vi "Kontroll Interferent Beschreibung Tabelle.vi"(4 "Sprachliste":string[][](array[string]), 6 "MFC-auswahl":T1 items=["MFC 2", "MFC 3", "MFC 4", "MFC 5"], 10 "Table Header":string[](array[string]), 11 "TestKonfig":T2 {"TestKonfig Interferent"."Gasflasche MFC3" items=["----"=10000, "IAG NH3 3000"=0, "IAG NH3 200"=1, "IAG NH3 2000"=2, "IAG MG"=3, "IAG O2"=4]; "TestKonfig Interferent"."Gasflasche MFC2" items=["----"=10000, "IAG NH3 3000"=0, "IAG NH3 200"=1, "IAG NH3 2000"=2, "IAG MG"=3, "IAG O2"=4]; "TestKonfig Interferent"."Eingangs Konzentration MFC1" min=0.0; "TestKonfig Interferent"."Ausgangs Konzentration MFC1" min=0.0; "TestKonfig Interferent"."MFC2" items=["MFC 2", "MFC 3", "MFC 4", "MFC 5"]; "TestKonfig Interferent"."MFC3" items=["MFC 2", "MFC 3", "MFC 4", "MFC 5"]; "TestKonfig Interferent"."Ausgangs Konzentration MFC3" min=0.0; "TestKonfig Interferent"."Eingangs Konzentration MFC3" min=0.0; "TestKonfig Interferent"."Ausgangs Konzentration MFC2" min=0.0; "TestKonfig Interferent"."Eingangs Konzentration MFC2" min=0.0; "TestKonfig H2O"."HovaCAL Temperature" format="%.2f"; "TestKonfig H2O"."HovaCAL Flow Input Cluster"."HovaCAL Flow Input Cluster" format="%.2f"; "TestKonfig H2O"."Eingangs Konzentration:" min=0.0; "TestKonfig H2O"."zusätzliche Zeitdauer Erster Punkt" min=30 step=1 format="%#_5g"; "TestKonfig H2O"."Zeitdauer Stufen" format="%#_5g"; "TestKonfig H2O"."Max Fehler" format="%#_5g"; "TestKonfig H2O"."Anzahl Stufen" format="%#_5g"; "TestKonfig H2O"."Modus" items=["Messen", "CG zu Entnahmestelle"]}) -> (3 "Tabelle":string[][](array[string]))   [LabVIEW 2020, in "EPA 1065.lvlib" / "HovaCAL Interference verificaton.lvlib"]
uses:
  HovaCAL Interference verificaton.lvlib
  TestKonfig.ctl
  TestKonfig H2O.ctl
  Modus.ctl
  Linearisierung V2/SpanEinstellungen/Einheit.ctl
  Linearisierung V2/Gasteiler/Stufen Tabelle.ctl
  Linearisierung V2/Gasteiler/HovaCAL_Interface/Controls/Flow Einstellung.ctl
  Linearisierung V2/Gasteiler/HovaCAL_Interface/Controls/Temp Sollwerte Anzeige.ctl
  TestKonfig Interferents.ctl
  MFCAuswahl.ctl
  Seiten/System Einstellungen V2/Gasflasche Auswahl.ctl
  Sprachverwaltung/Sprachverwaltung.lvlib
  Linearisierung V2/SpanEinstellungen/SpanEinstellungen.lvlib
  Linearisierung V2/Gasteiler/Gasteiler.lvlib
  Linearisierung V2/Gasteiler/HovaCAL_Interface/Controls/Controls.lvlib
  Seiten/System Einstellungen V2/System Einstellungen V2.lvlib
panel:
  # "sec"
  # "%"
  # "sec"
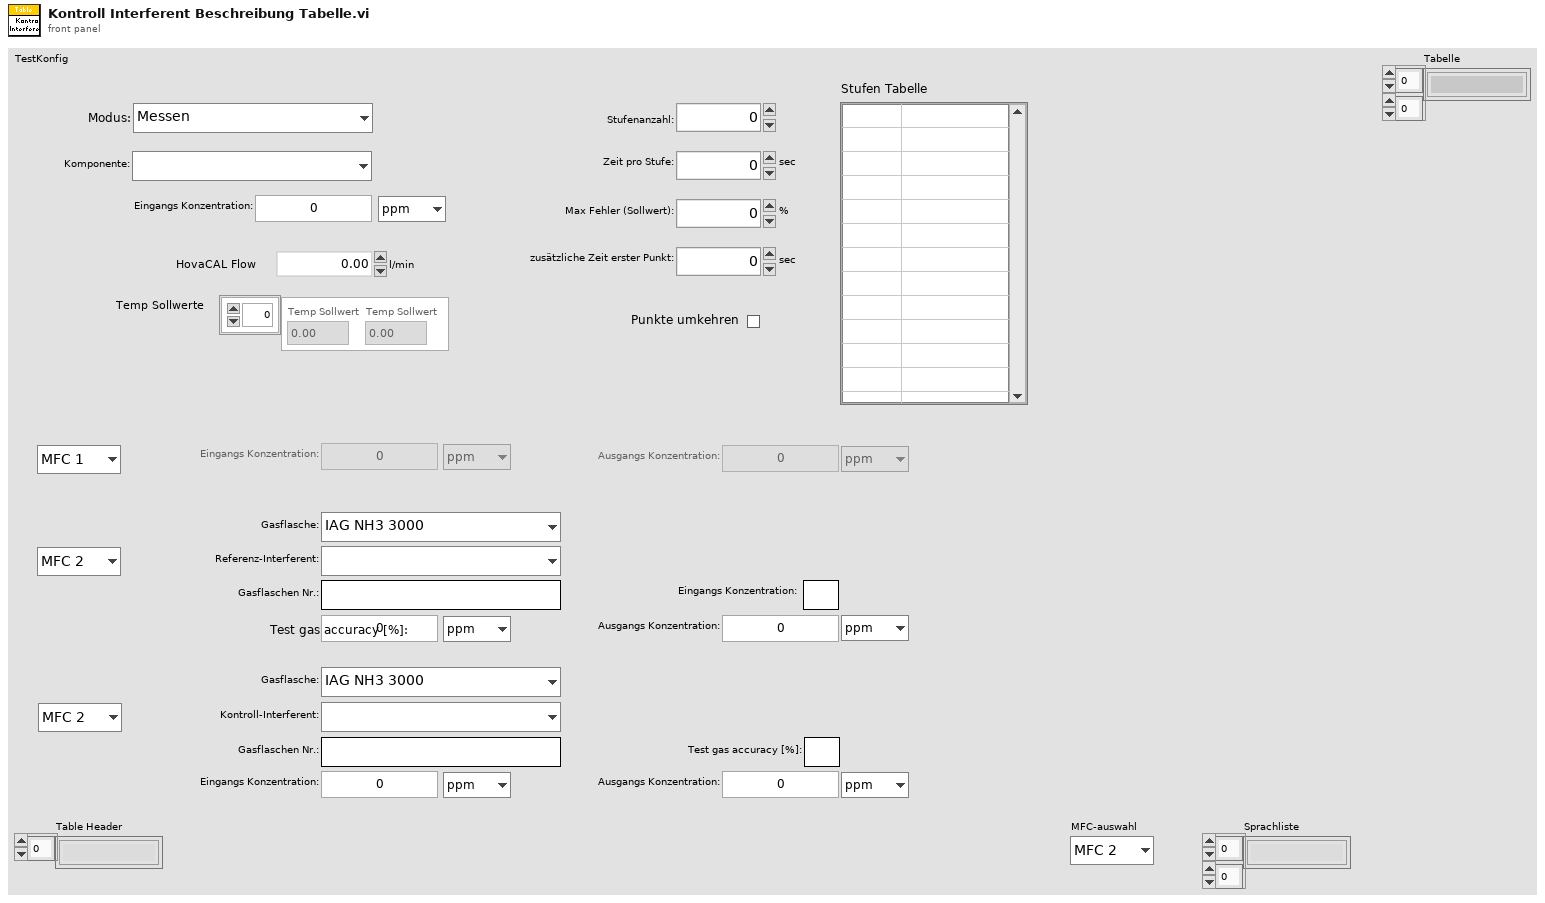
[diagram p1: front panel]
types:
  T1 = typedef "EPA 1065.lvlib/HovaCAL Interference verificaton.lvlib/MFCAuswahl.ctl" = u16
  T2 = typedef "EPA 1065.lvlib/HovaCAL Interference verificaton.lvlib/TestKonfig.ctl" = cluster{"TestKonfig H2O":T3, "TestKonfig Interferent":T9}
  T3 = typedef "EPA 1065.lvlib/HovaCAL Interference verificaton.lvlib/TestKonfig H2O.ctl" = cluster{"Modus":T4, "Komponente:":u16, "Eingangs Konzentration:":dbl, "Einheit":T5, "Anzahl Stufen":sgl, "Zeitdauer Stufen":sgl, "Max Fehler":sgl, "zusätzliche Zeitdauer Erster Punkt":sgl, "Punkte umkehren":bool, "Stufen Tabelle":T6, "HovaCAL Flow Input Cluster":T7, "HovaCAL Temperature":T8}
  T4 = typedef "EPA 1065.lvlib/HovaCAL Interference verificaton.lvlib/Modus.ctl" = u16
  T5 = typedef "Linearisierung v2.lvlib/SpanEinstellungen.lvlib/Einheit.ctl" = enum16{"ppm", "%"}
  T6 = typedef "Linearisierung v2.lvlib/Gasteiler.lvlib/Stufen Tabelle.ctl" = string[][]
  T7 = typedef "Linearisierung v2.lvlib/Gasteiler.lvlib/HovaCAL_Interface.lvlib/Controls.lvlib/Flow Einstellung.ctl" = cluster{"HovaCAL Flow Input Cluster":dbl}
  T8 = typedef "Linearisierung v2.lvlib/Gasteiler.lvlib/HovaCAL_Interface.lvlib/Controls.lvlib/Temp Sollwerte Anzeige.ctl" = dbl[]
  T9 = typedef "EPA 1065.lvlib/HovaCAL Interference verificaton.lvlib/TestKonfig Interferents.ctl" = cluster{"MFC1":enum16{"MFC 1"}, "Eingangs Konzentration MFC1":dbl, "Einheit MFC1 Eingang":T5, "Ausgangs Konzentration MFC1":dbl, "Einheit MFC1 Ausgang":T5, "MFC2":T1, "Referenz-Interferent:":u16, "Gasflaschen Nr MFC2":string, "Accuracy MFC2":string, "Eingangs Konzentration MFC2":dbl, "Einheit MFC2 Eingang":T5, "Ausgangs Konzentration MFC2":dbl, "Einheit MFC2 Ausgang":T5, "MFC3":T1, "Kontroll-Interferent:":u16, "Gasflaschen Nr MFC3":string, "Accuracy MFC3":string, "Eingangs Konzentration MFC3":dbl, "Einheit MFC3 Eingang":T5, "Ausgangs Konzentration MFC3":dbl, "Einheit MFC3 Ausgang":T5, "Gasflasche MFC2":T10, "Gasflasche MFC3":T10}
  T10 = typedef "System Einstellungen V2.lvlib/Gasflasche Auswahl.ctl" = u16
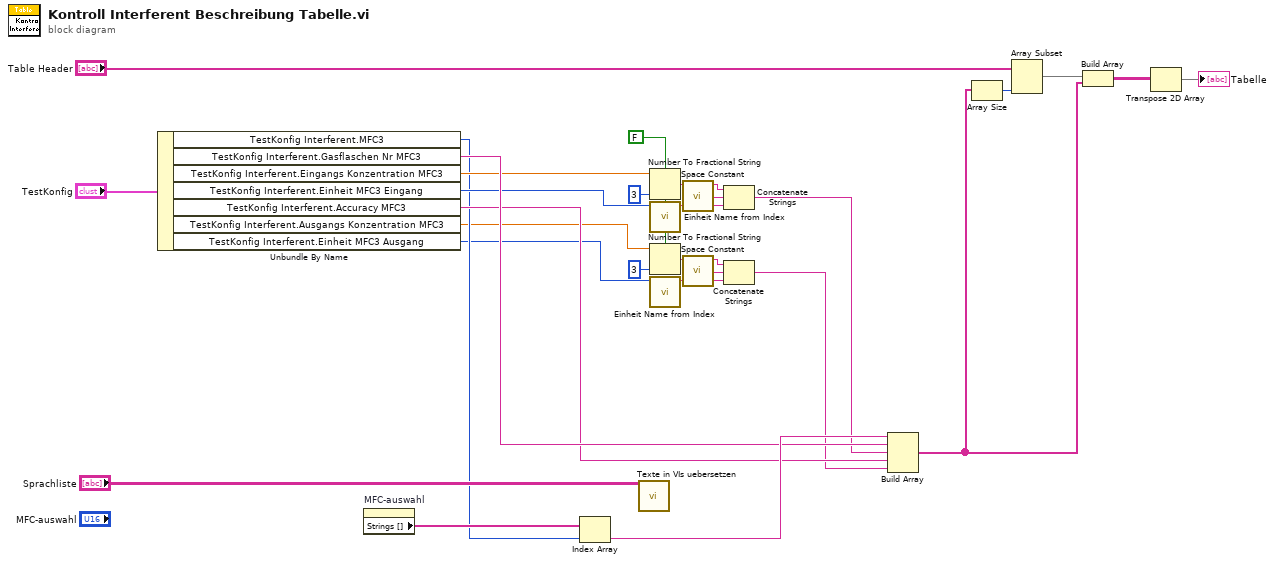
[diagram p0: block diagram]
diagram:
  w8 = FALSE ("Systemdezimalzeichen verwenden (T)")
  n1 = Unbundle By Name("TestKonfig") -> ("TestKonfig Interferent.MFC3"=w13:T1, "TestKonfig Interferent.Gasflaschen Nr MFC3"=w18:string, "TestKonfig Interferent.Eingangs Konzentration MFC3"=w17:dbl, "TestKonfig Interferent.Einheit MFC3 Eingang"=w15:T5, "TestKonfig Interferent.Accuracy MFC3"=w14:string, "TestKonfig Interferent.Ausgangs Konzentration MFC3"=w7:dbl, "TestKonfig Interferent.Einheit MFC3 Ausgang"=w6:T5)
  n2 = property on="MFC-auswahl" class="Ring (strikt)"() -> ("Strings []"=w20:string[])  [unwired: 2 in, 2 out]
  n3 = Index Array(array=w20, index=w13) -> (element=w19:string)
  n4 = call "Texte in VIs uebersetzen.vi"("Sprachliste"="Sprachliste") -> ()  [unwired: 10 in, 5 out]
  n5 = Number To Fractional String(use system decimal point (T)=w8, number=w17, precision (6)=i16 3 ("Genauigkeit (6)")) -> (F-format string=w23:string)  [unwired: 1 in]
  n6 = call "Einheit Name from Index.vi"("EinheitIndex"=w15) -> ("EinheitName"=w24:string)  [unwired: 10 in]
  n7 = Number To Fractional String(use system decimal point (T)=w8, number=w7, precision (6)=i16 3 ("Genauigkeit (6)")) -> (F-format string=w11:string)  [unwired: 1 in]
  n8 = call "Einheit Name from Index.vi"("EinheitIndex"=w6) -> ("EinheitName"=w10:string)  [unwired: 10 in]
  n9 = call <vilib>:"Space Constant.vi"() -> ("String"=w22:string)
  n10 = call <vilib>:"Space Constant.vi"() -> ("String"=w12:string)
  n11 = Concatenate Strings(w23, w22, w24) -> (w16:string)
  n12 = Concatenate Strings(w11, w12, w10) -> (w5:string)
  n13 = Build Array(w19, w18, w16, w14, w5) -> (w4:string[])
  n14 = Array Size(array=w4) -> (size(s)=w2:i32)
  n15 = Array Subset(array="Table Header", length=w2) -> (w1:string[])  [unwired: 1 in]
  n16 = Build Array(w1, w4) -> (w26:string[][])
  n17 = Transpose 2D Array(2D array=w26) -> (transposed array=→"Tabelle":string[][])
